vi "Begin.vi"(8 "error in":errorcluster) -> (0 "error out":errorcluster)   [LabVIEW 2017]
doc: "Called before other user functions, this VI can be used to open I/O refnums, load in file data, and do general program initialization. Notice that the <B>error out</B> terminal is simply used for data flow. Wiring it to other structures or subVIs ensures that this VI runs first."
uses:
  <vilib>/Rock Robotics/WPI/DriverStation/WPI_DriverStationRobotMode2.ctl
  <vilib>/Rock Robotics/WPI/Joystick/WPI_JoystickDeviceEnum.ctl
  Logging/LogOperation.ctl
  Robot Global Data.vi
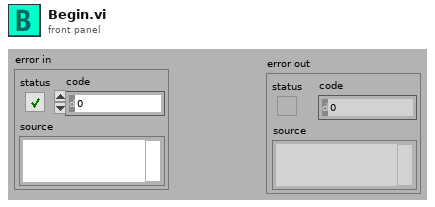
[diagram p1: front panel]
types:
  T1 = typedef "LogOperation.ctl" = enum16{"Set", "Get All", "Init"}
  T2 = typedef "WPI_JoystickDeviceEnum.ctl" = enum16{"USB 0", "USB 1", "USB 2", "USB 3", "USB 4", "USB 5"}
  T3 = typedef "WPI_DriverStationRobotMode2.ctl" = enum16{"Autonomous Disabled", "Autonomous Enabled", "Teleop Disabled", "Teleop Enabled", "Disconnected", "Finish", "Test Disabled", "Test Enabled", "Emergency Stopped"}
  T4 = typedef "WPI_JoystickDevRef.ctl" = cluster{"Device":T2}
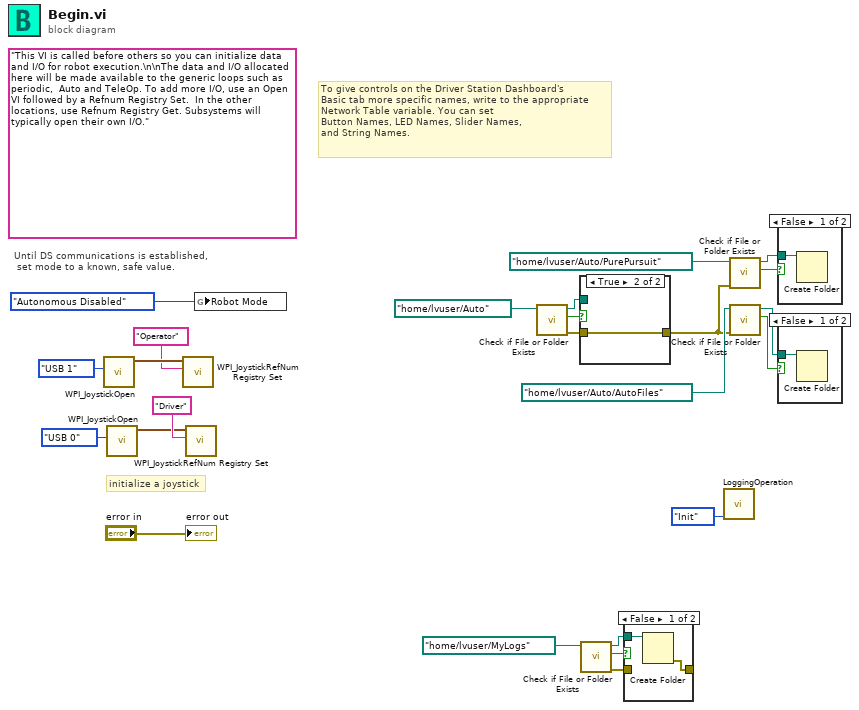
[diagram p0: block diagram]
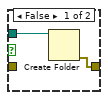
[diagram p5: hidden frame]
diagram:
  (unwired) "This VI is called before others so you can initialize data and I/O for robot execution.\n\nThe data and I/O allocated here will be made available to the generic loops such as periodic,  Auto and TeleOp. To add more I/O, use an Open VI followed by a Refnum Registry Set.  In the other locations, use Refnum Registry Get. Subsystems will typically open their own I/O."
  # "To give controls on the Driver Station Dashboard's\nBasic tab more specific names, write to the appropriate\nNetwork Table variable. You can set\nButton Names, LED Names, Slider Names,\nand String Names."
  # "initialize a joystick"
  # "Until DS communications is established,\n set mode to a known, safe value."
  n1 = call <vilib>:"WPI_JoystickOpen.vi"("JoystickDevice"=WPI_JoystickDeviceEnum."USB 1") -> ("JoystickDevRef"=w3:T4)  [unwired: 10 in]
  n2 = call <vilib>:"WPI_JoystickOpen.vi"("JoystickDevice"=WPI_JoystickDeviceEnum."USB 0") -> ("JoystickDevRef"=w22:T4)  [unwired: 10 in]
  n3 = call <vilib>:"WPI_JoystickRefNum Registry Set.vi"("refnum name"="Operator", "JoystickDevRef"=w3) -> ()  [unwired: 8 in, 2 out]
  n4 = call <vilib>:"WPI_JoystickRefNum Registry Set.vi"("refnum name"="Driver", "JoystickDevRef"=w22) -> ()  [unwired: 8 in, 2 out]
  n5 = global write "Robot Global Data.vi" "Robot Mode"(WPI_DriverStationRobotMode2."Autonomous Disabled" ("Robot Mode")) -> ()
  n6 = call <vilib>:"Check if File or Folder Exists.vi"("path"=path "/home/lvuser/Auto") -> ("error out"=w19:errorcluster, "file or folder exists?"=w18:bool, "dup path"=w17:path)  [unwired: 8 in]
  n7 = case shown="True" w18 {
    tunnel: w17 -> [w26 _]
    tunnel: [w25 w27] -> w9
    tunnel: w19 -> [_ w27]
    frame False {
      n8 = Create Folder(path (use dialog)=w26) -> (error out=w25:errorcluster)  [unwired: 2 in, 2 out]
    }
    frame True {
    }
  }
  n9 = call <vilib>:"Check if File or Folder Exists.vi"("path"=path "/home/lvuser/MyLogs") -> ("error out"=w8:errorcluster, "file or folder exists?"=w7:bool, "dup path"=w6:path)  [unwired: 8 in]
  n10 = case shown="False" w7 {
    tunnel: w6 -> [w29 _]
    tunnel: [w28 w30] -> _
    tunnel: w8 -> [_ w30]
    frame False {
      n11 = Create Folder(path (use dialog)=w29) -> (error out=w28:errorcluster)  [unwired: 2 in, 2 out]
    }
    frame True {
    }
  }
  n12 = call "LoggingOperation.vi"("Operation"=LogOperation."Init") -> ()  [unwired: 10 in, 1 out]
  n13 = call <vilib>:"Check if File or Folder Exists.vi"("error in (no error)"=w9, "path"=path "/home/lvuser/Auto/PurePursuit") -> ("file or folder exists?"=w15:bool, "dup path"=w14:path)  [unwired: 7 in, 1 out]
  n14 = call <vilib>:"Check if File or Folder Exists.vi"("error in (no error)"=w9, "path"=path "/home/lvuser/Auto/AutoFiles") -> ("file or folder exists?"=w11:bool, "dup path"=w12:path)  [unwired: 7 in, 1 out]
  n15 = case shown="False" w15 {
    tunnel: w14 -> [w31 _]
    frame False {
      n16 = Create Folder(path (use dialog)=w31) -> ()  [unwired: 2 in, 3 out]
    }
    frame True {
    }
  }
  n17 = case shown="False" w11 {
    tunnel: w12 -> [w32 _]
    frame False {
      n18 = Create Folder(path (use dialog)=w32) -> ()  [unwired: 2 in, 3 out]
    }
    frame True {
    }
  }
  "error out" <- "error in"
